vi "Configure Flow Deceleration.vi"(7 "Pump ID (0:A)":T1, 8 "error in (no error)":errorcluster, 10 "Flow Deceleration  (500 uL/s^2)":dbl=500.0, 11 "VISA resource in":refnum<visa-resource-name>) -> (0 "error out":errorcluster, 3 "VISA resource out":refnum<visa-resource-name>)   [LabVIEW 2020, in "Global FIA milliGAT.lvlib"]
doc: "Configuration the motion settings:; initial flow rate, acceleration, deceleration, and max flow rate."
uses:
  <instrlib>/RxnRover/Global FIA milliGAT 3.14/Global FIA milliGAT.lvlib
  <instrlib>/RxnRover/Global FIA milliGAT 3.14/Public/Utility/Pump Address.ctl
  <instrlib>/RxnRover/Global FIA milliGAT 3.14/Private/Pump Parameter.ctl
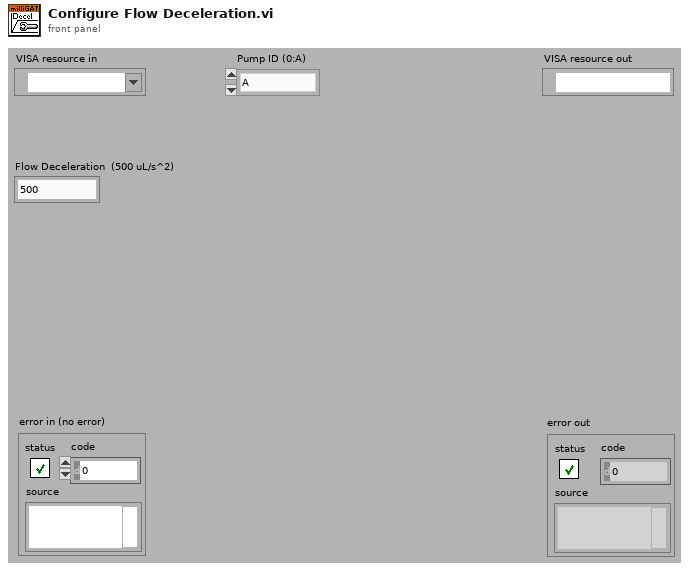
[diagram p1: front panel]
types:
  T1 = typedef "Global FIA milliGAT.lvlib/Pump Address.ctl" = enum16{"A", "B", "C", "D", "E", "F", "G", "H", "I", "J", "K", "L", "M", "N", "O", "P", "Q", "R", "S", "T", "U", "V", "W", "X", "Y", "Z", "a", "b", "c", "d", "e", "f", "g", "h", "i", "j", "k", "l", "m", "n", "o", "p", "q", "r", "s", "t", "u", "v", "w", "x", "y", "z", "0", "1", "2", "3", "4", "5", "6", "7", "8", "9"}
  T2 = typedef "Global FIA milliGAT.lvlib/Pump Parameter.ctl" = enum16{"Enabled", "EU", "EU Calibration Factor", "Fixed Asp or Disp", "Starting Position", "Starting Flow", "Peak Flow", "Flow Acceleration", "Flow Deceleration", "Session Volume", "Max Pressure", "Backlash (usteps)", "BL Calibration Factor", "BL Correction Enabled", "Min Flow", "Max Flow", "Min Acceleration", "Max Acceleration", "Service Volume", "Life Volume"}
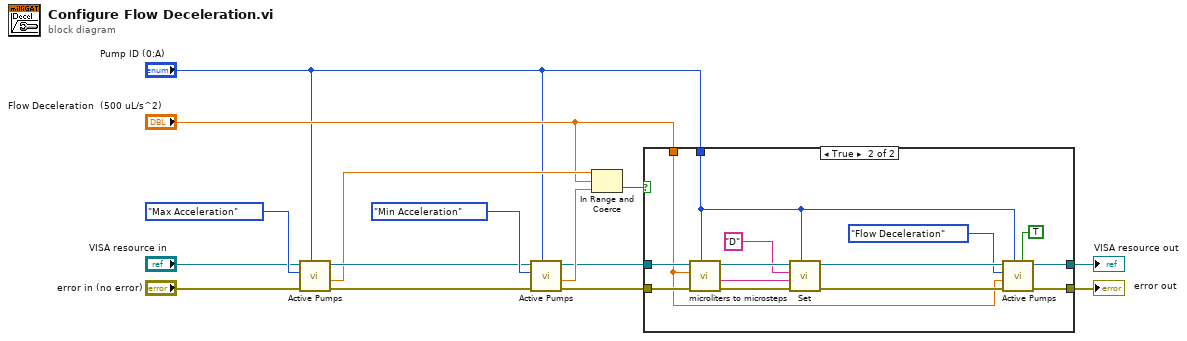
[diagram p0: block diagram]
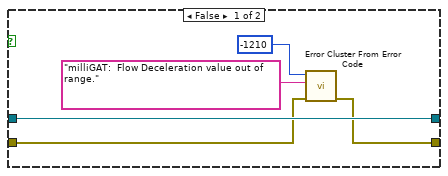
[diagram p2: hidden frame]
diagram:
  n1 = call <instrlib>:"Active Pumps.vi"("Pump ID (0:A)"="Pump ID (0:A)", "error in (no error)"="error in (no error)", "Parameter"=Pump_Parameter."Max Acceleration", "VISA resource in"="VISA resource in") -> ("error out"=w10:errorcluster, "Value out"=w9:dbl, "VISA resource out"=w11:refnum<visa-resource-name>)  [unwired: 4 in, 1 out]
  n2 = call <instrlib>:"Active Pumps.vi"("Pump ID (0:A)"="Pump ID (0:A)", "error in (no error)"=w10, "Parameter"=Pump_Parameter."Min Acceleration", "VISA resource in"=w11) -> ("error out"=w5:errorcluster, "Value out"=w8:dbl, "VISA resource out"=w4:refnum<visa-resource-name>)  [unwired: 4 in, 1 out]
  n3 = In Range and Coerce(upper limit=w9, x="Flow Deceleration  (500 uL/s^2)", lower limit=w8) -> (In Range?=w3:bool)  [unwired: 1 out]
  n4 = case shown="True" w3 {
    tunnel: w4 -> [w20 w34]
    tunnel: w5 -> [w17 w33]
    tunnel: [w16 w25] -> w2
    tunnel: [w20 w26] -> w1
    tunnel: "Pump ID (0:A)" -> [_ w24]
    tunnel: "Flow Deceleration  (500 uL/s^2)" -> [_ w21]
    frame False {
      n5 = call <vilib>:"Error Cluster From Error Code.vi"("error in (no error)"=w17, "error message (\"\")"="milliGAT:  Flow Deceleration value out of range." ("error message (\"\")"), "error code (0)"=-1210) -> ("error out"=w16:errorcluster)  [unwired: 6 in]
    }
    frame True {
      n6 = call <instrlib>:"microliters to microsteps.vi"("Pump ID (0:A)"=w24, "error in (no error)"=w33, "Microliters (0)"=w21, "VISA resource in"=w34) -> ("error out"=w31:errorcluster, "Microsteps (STR)"=w30:string, "VISA resource out"=w32:refnum<visa-resource-name>)  [unwired: 4 in, 1 out]
      n7 = call <instrlib>:"Set.vi"("Pump ID (0:A)"=w24, "error in (no error)"=w31, "Expression"=w30, "Parameter"="D", "VISA resource in"=w32) -> ("error out"=w27:errorcluster, "VISA resource out"=w28:refnum<visa-resource-name>)  [unwired: 5 in]
      n8 = call <instrlib>:"Active Pumps.vi"("Action (F:Read)"=TRUE, "Pump ID (0:A)"=w24, "error in (no error)"=w27, "Value in"=w21, "Parameter"=Pump_Parameter."Flow Deceleration", "VISA resource in"=w28) -> ("error out"=w25:errorcluster, "VISA resource out"=w26:refnum<visa-resource-name>)  [unwired: 2 in, 2 out]
    }
  }
  "VISA resource out" <- w1
  "error out" <- w2
